vi "test.vi"() -> ()   [LabVIEW 2013]
panel:
  in  "Trig now":bool
  in  "Software Trig":bool
  in  "stop":bool
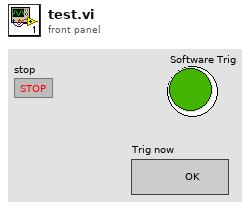
[diagram p1: front panel]
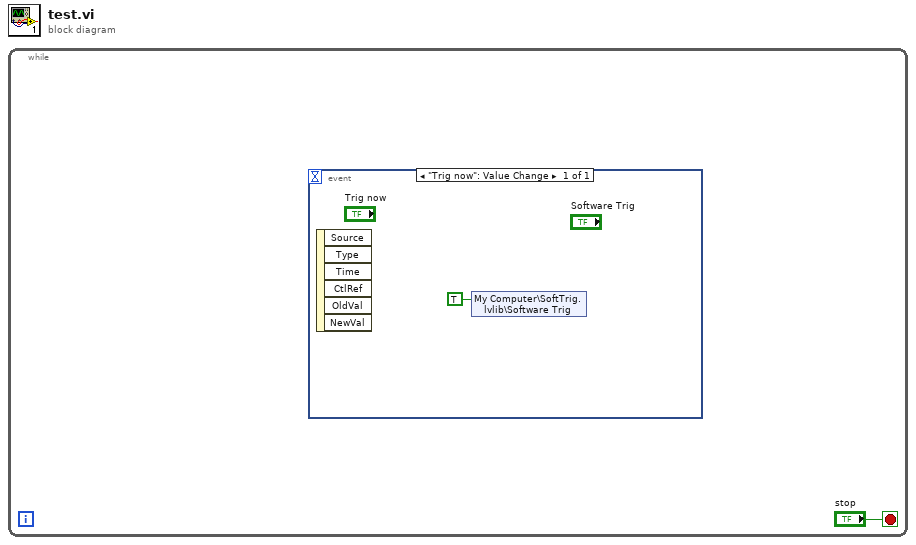
[diagram p0: block diagram]
diagram:
  n1 = while {
    stop <- "stop" stop-if-true
    n2 = event shown="[0] \"Trig now\": Value Change" {
      selector: _ -> [_]
      dyn-events: _ -> [_]
      timeout: _ -> [_]
      event "Trig now": Value Change {
        n3 = event-data() -> ()  [unwired: 1 in, 6 out]
        n4 = shared-variable "My Computer\\SoftTrig.lvlib\\Software Trig"(TRUE ("Software Trig")) -> ()  [unwired: 1 in, 1 out]
      }
    }
  }
